vi "tvac_gui_v3.vi"() -> ()   [LabVIEW 2017]
uses:
  <vilib>/httpClient/ClientHandle.ctl
  msg7171_linux.llb/send single message.vi
  <vilib>/httpClient/POSTBuffer.vi
  <vilib>/httpClient/LabVIEWHTTPClient.lvlib
panel:
  in  "index (col)":i32
  in  "alarm":i32
  in  "NumberTCs":i32=10
  in  "Tab Control":enum32{"Page 1", "Page 2"}(tab)
  in  "Zone 1":T1 {"Ring" items=["Average", "Maximum", "Minimum", ""]}
  in  "Graphing Selection":u16(ring) items=["User Selection", "Graph All Thermocouples", "Clear Graph"]
  in  "Time Scale":u16(ring) items=["Minutes", "Hours", "Seconds"]
  out "Waveform Chart":waveform(dbl)[](graph)
  out "Thermocouples":T2(array[cluster])
  in  "exit":bool
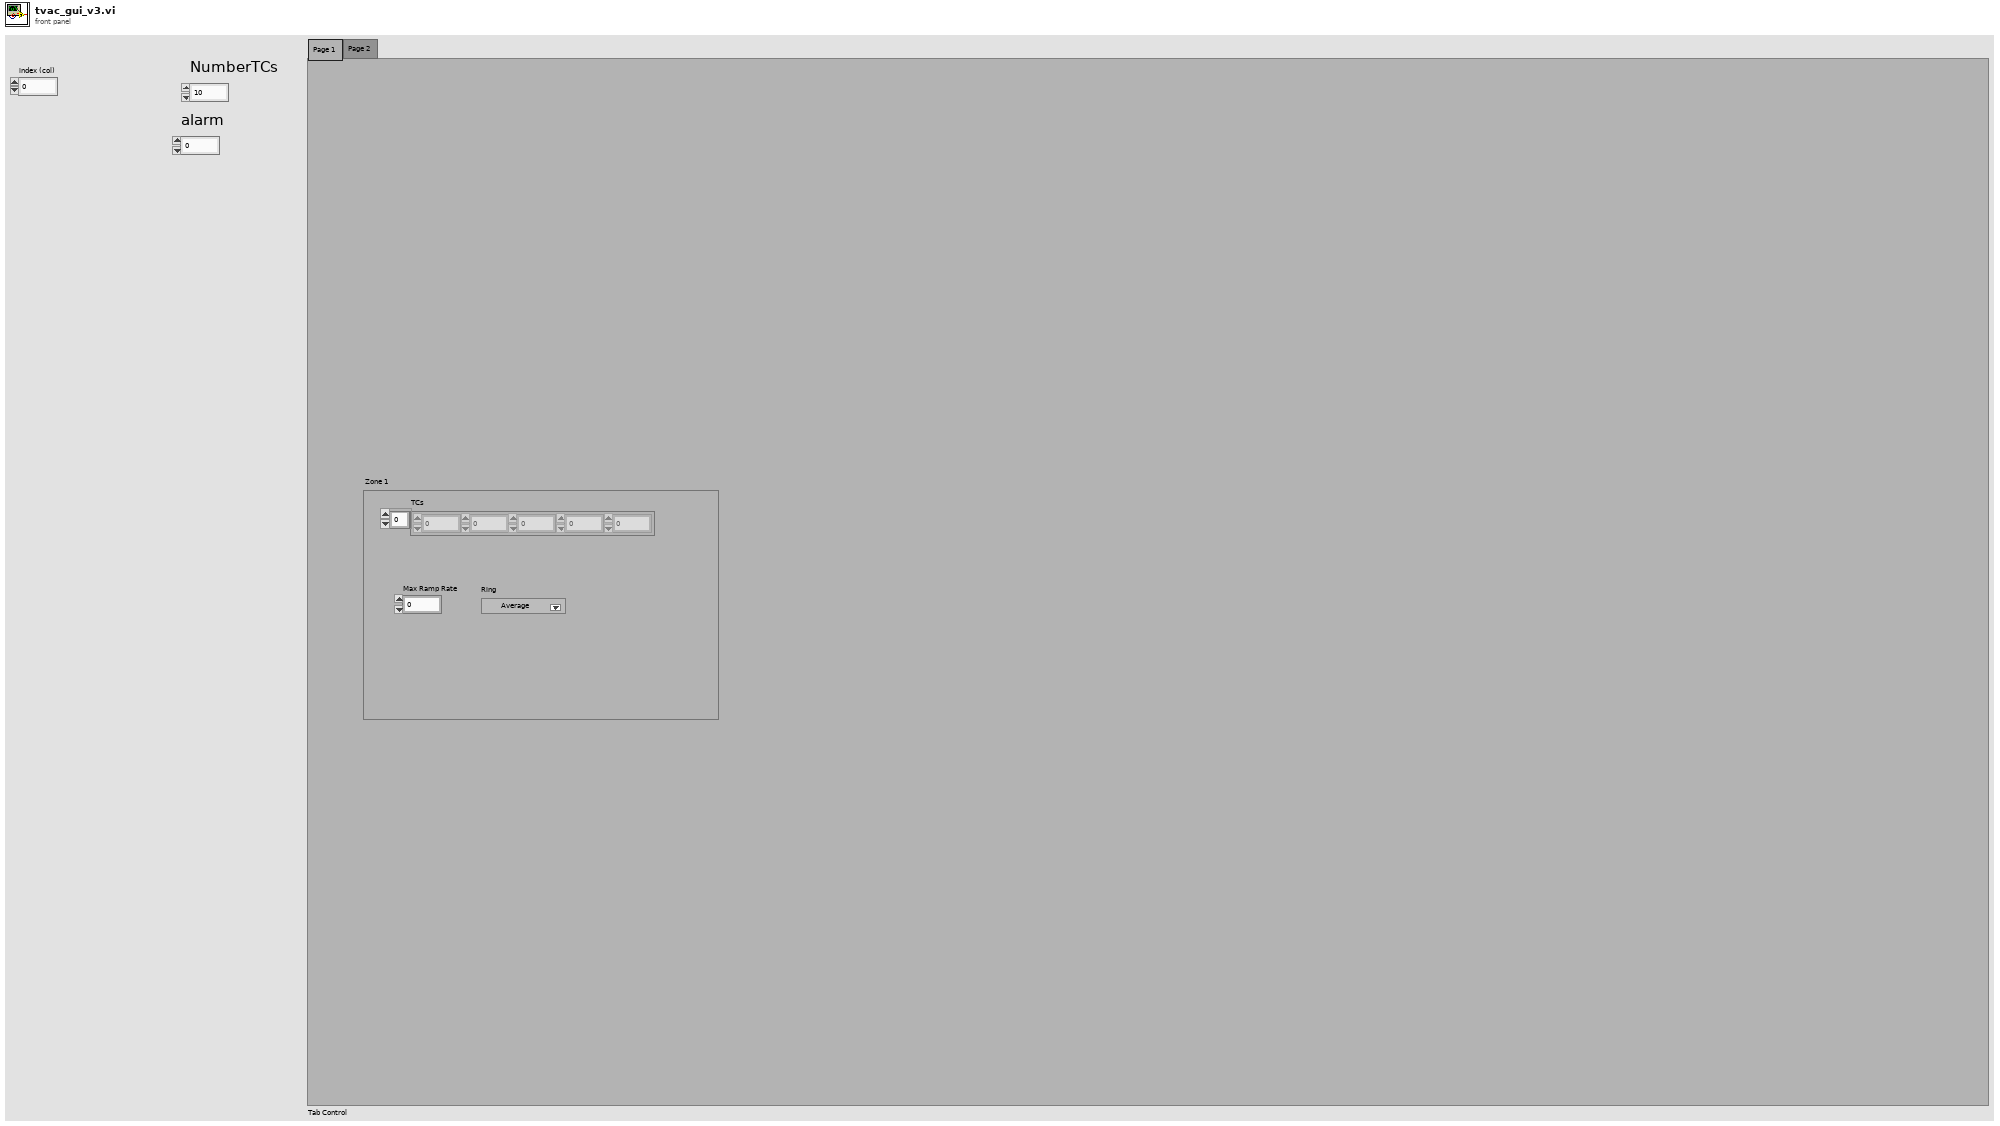
[diagram p1: front panel]
types:
  T1 = cluster{"Ring":u16, "Max Ramp Rate":dbl, "TCs":dbl[]}
  T2 = cluster{"TC Label":string, "Alarm Status":string, "Alarm Color":u32, "Temperature":string, "PlotColor":u32, "Graph On/Off":u32}[][]
  T3 = typedef "LabVIEWHTTPClient.lvlib/ClientHandle.ctl" = refnum<k1>
  T4 = cluster{"go":bool, "Http session":T3, "URL prefex":string}
  T5 = typedef "LVPoint32TypeDef.ctl" = cluster{"Horizontal":i32, "Vertical":i32}
  T6 = typedef "LVPositionTypeDef.ctl" = cluster{"Left":i32, "Top":i32}
  T7 = cluster{"TC Label":string, "Alarm Status":string, "Alarm Color":u32, "Temperature":string, "PlotColor":u32, "Graph On/Off":u32}
  T8 = typedef "LVRangeTypeDef.ctl" = cluster{"Minimum":dbl, "Maximum":dbl, "Increment":dbl, "Minor Increment":dbl, "Start":dbl}
  T9 = cluster{"time":string, "tcs":cluster{"thermocouple":i32, "time":i32, "temp":i32, "working":string, "alarm":i32}[]}
  T10 = cluster{"time":string, "tcs":cluster{"thermocouple":i32, "time":i32, "temp":i32, "working":i32, "alarm":i32}[]}
  T11 = cluster{"thermocouple":i32, "time":i32, "temp":i32, "working":i32, "alarm":i32}[]
  T12 = cluster{"thermocouple":i32, "time":i32, "temp":i32, "working":i32, "alarm":i32}
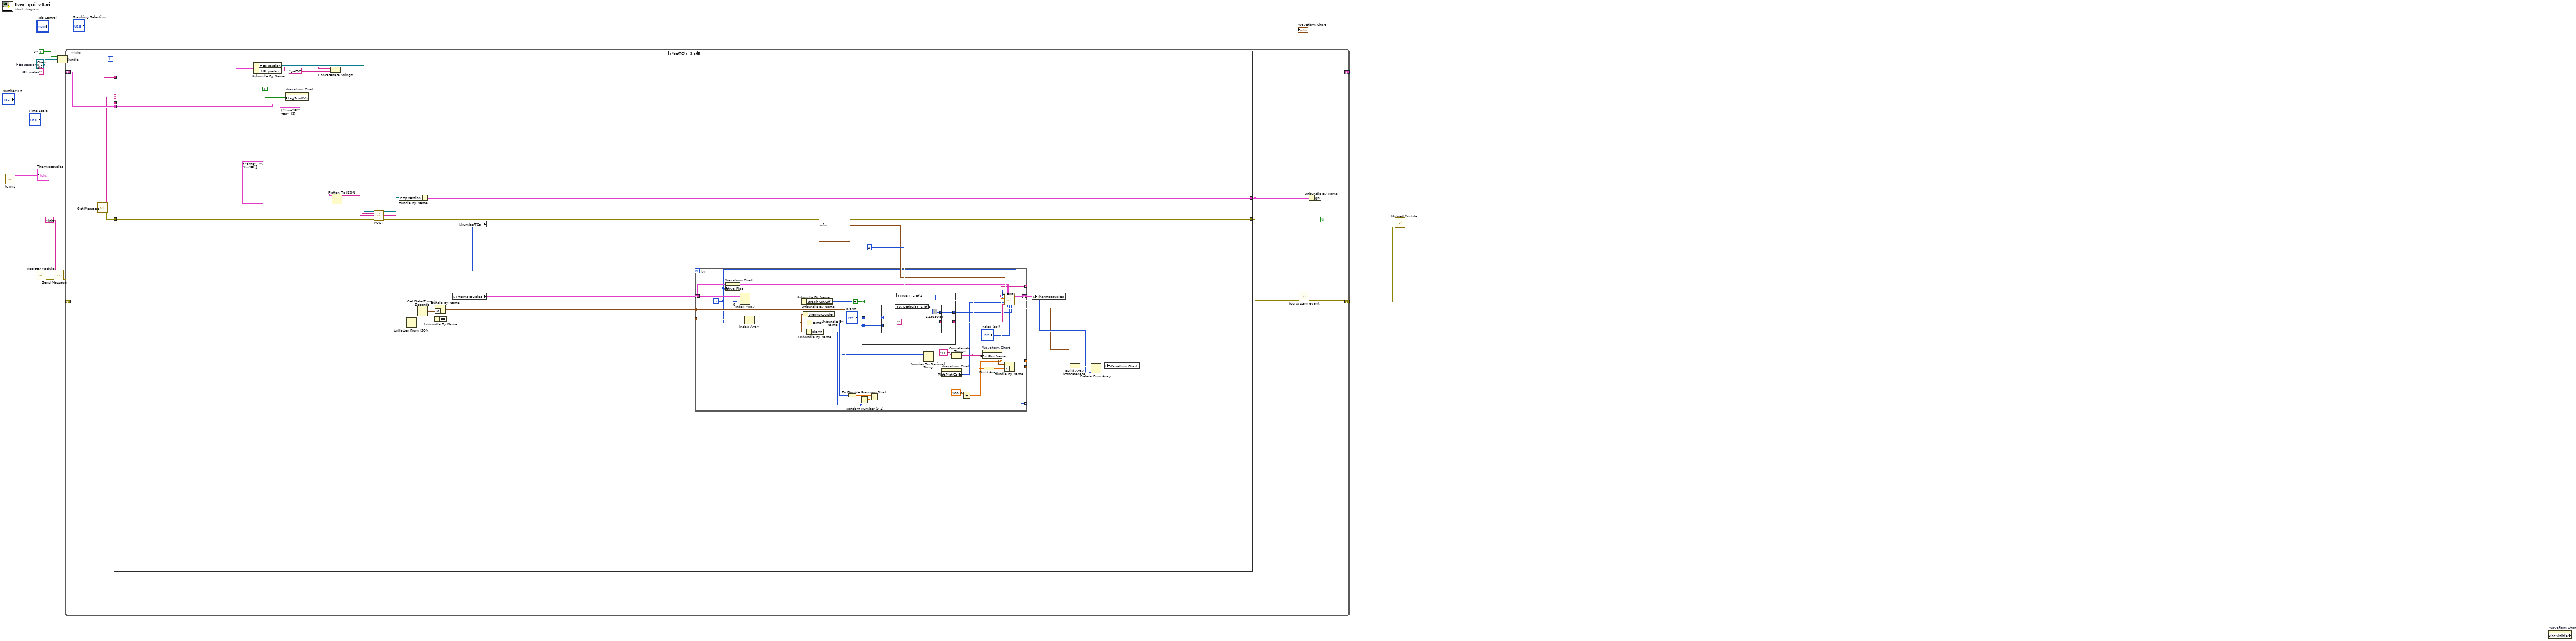
[diagram p0: block diagram]
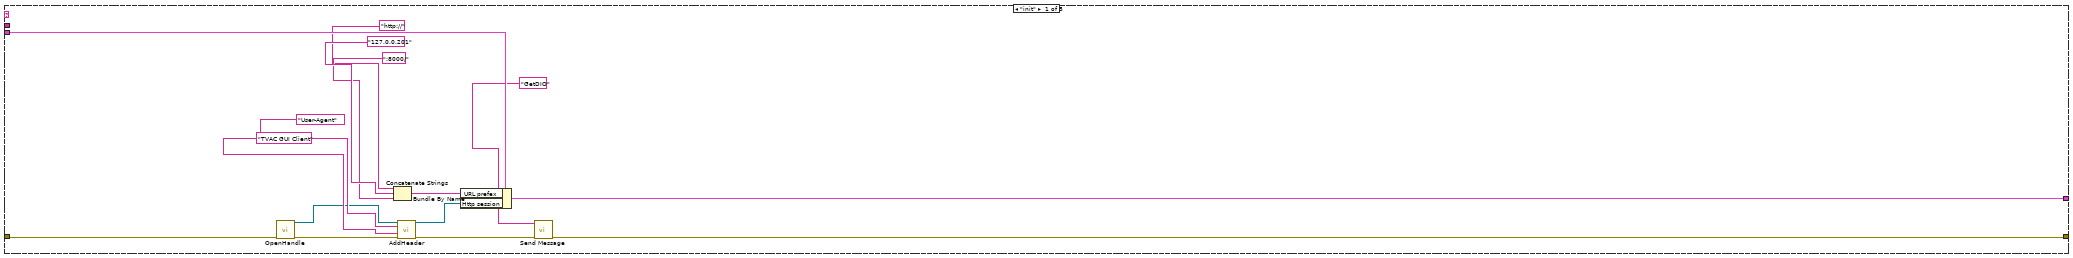
[diagram p2: hidden frame]
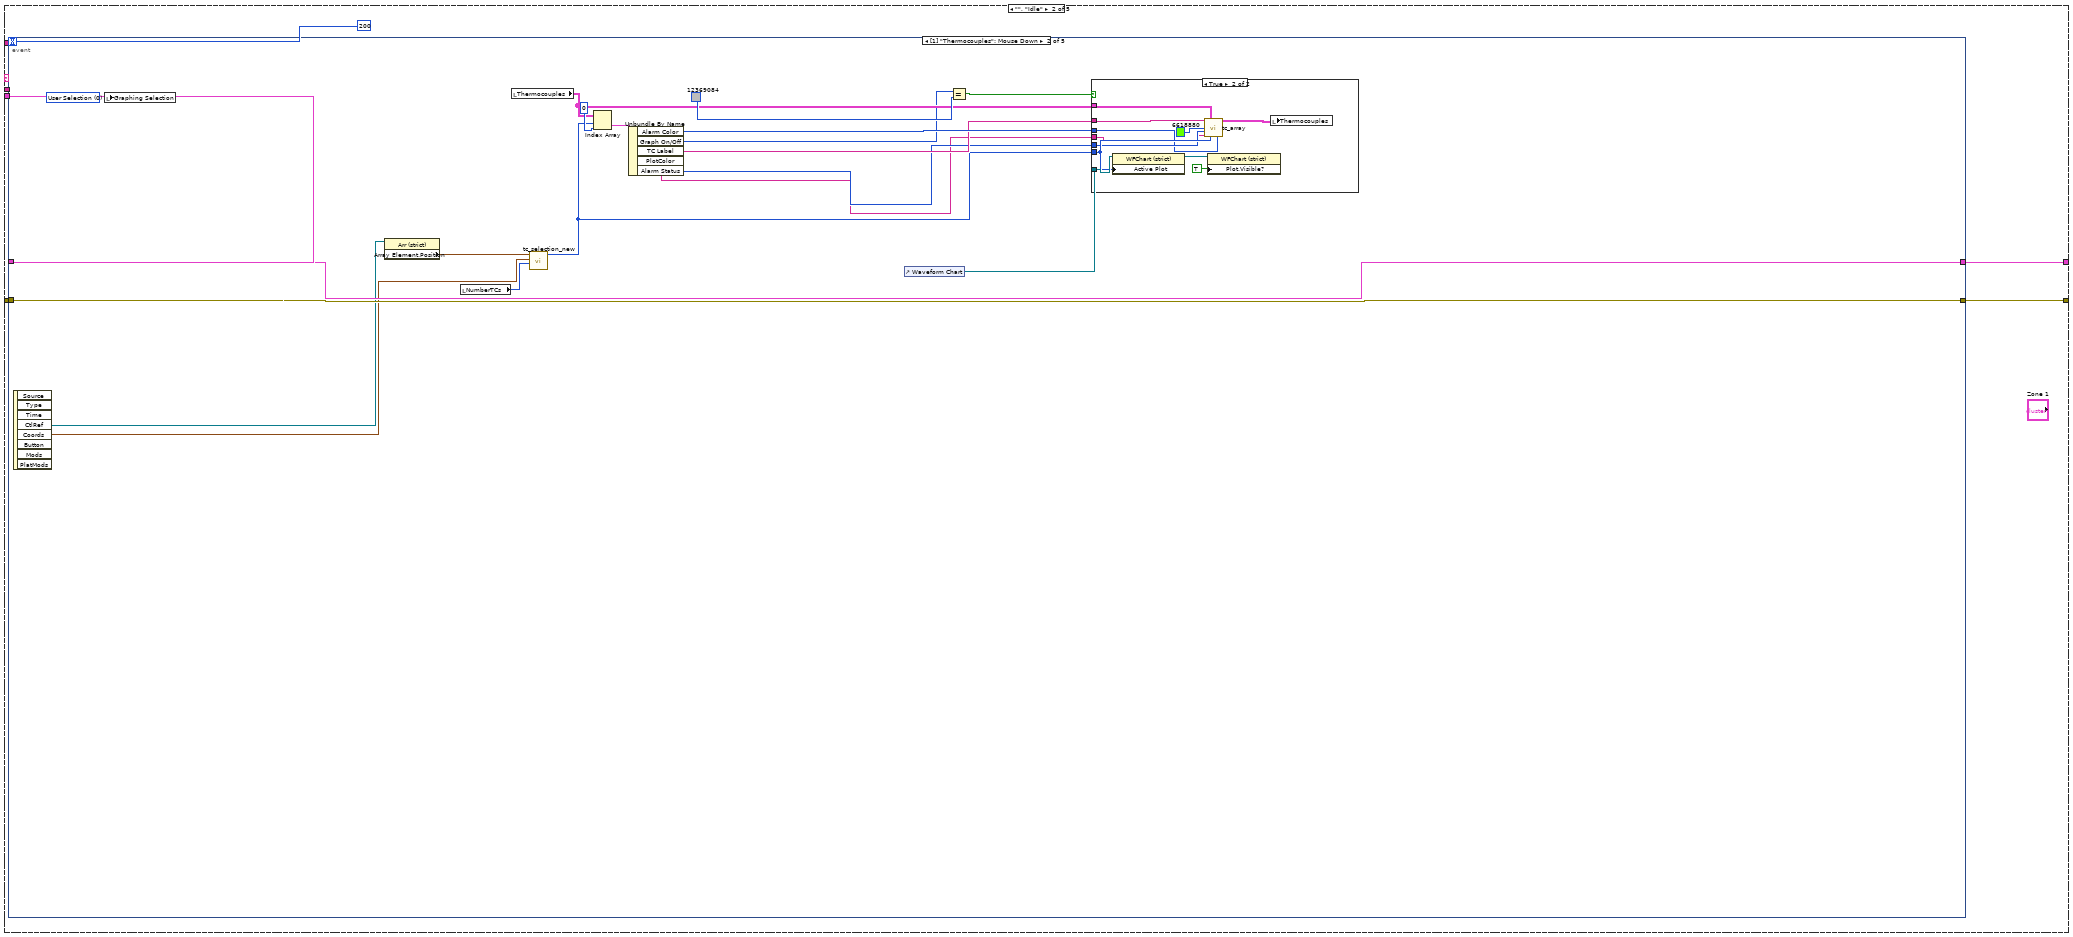
[diagram p3: hidden frame]
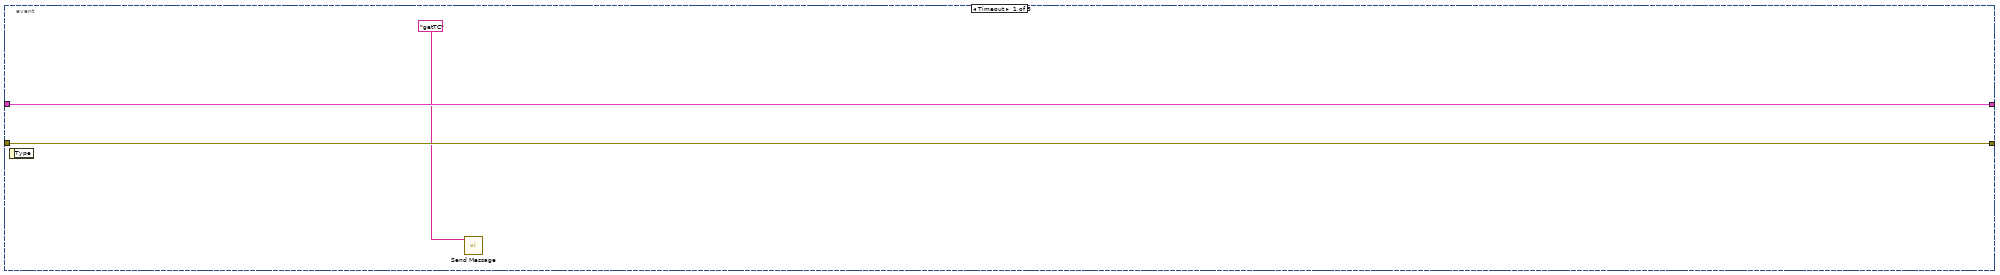
[diagram p4: hidden frame]
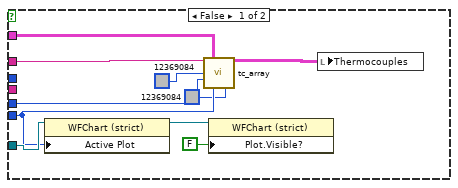
[diagram p5: hidden frame]
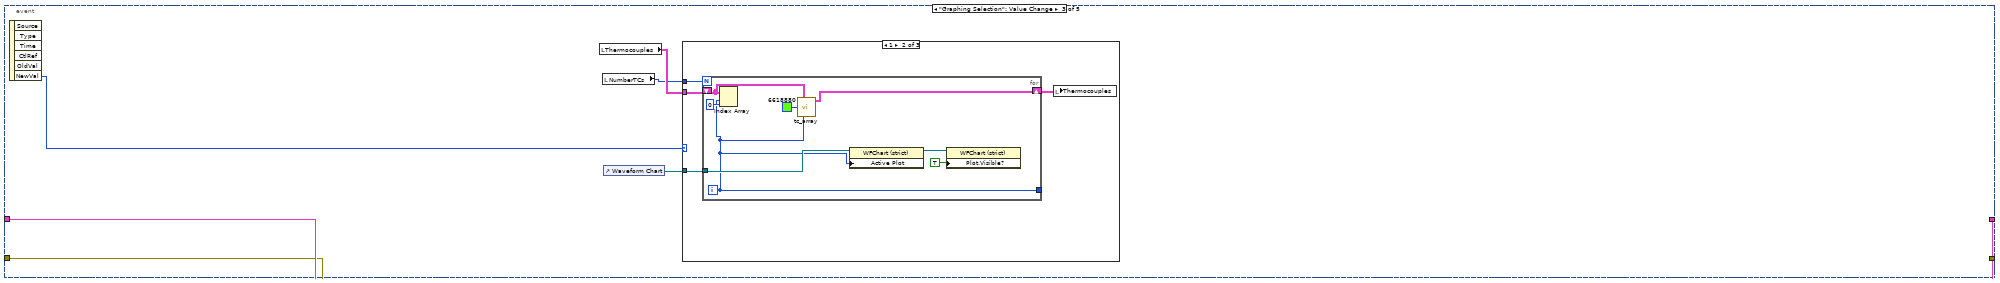
[diagram p6: hidden frame]
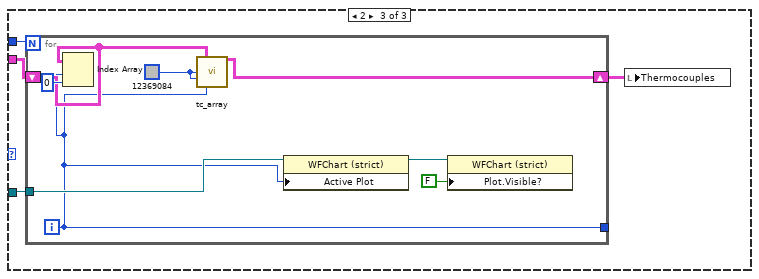
[diagram p8: hidden frame]
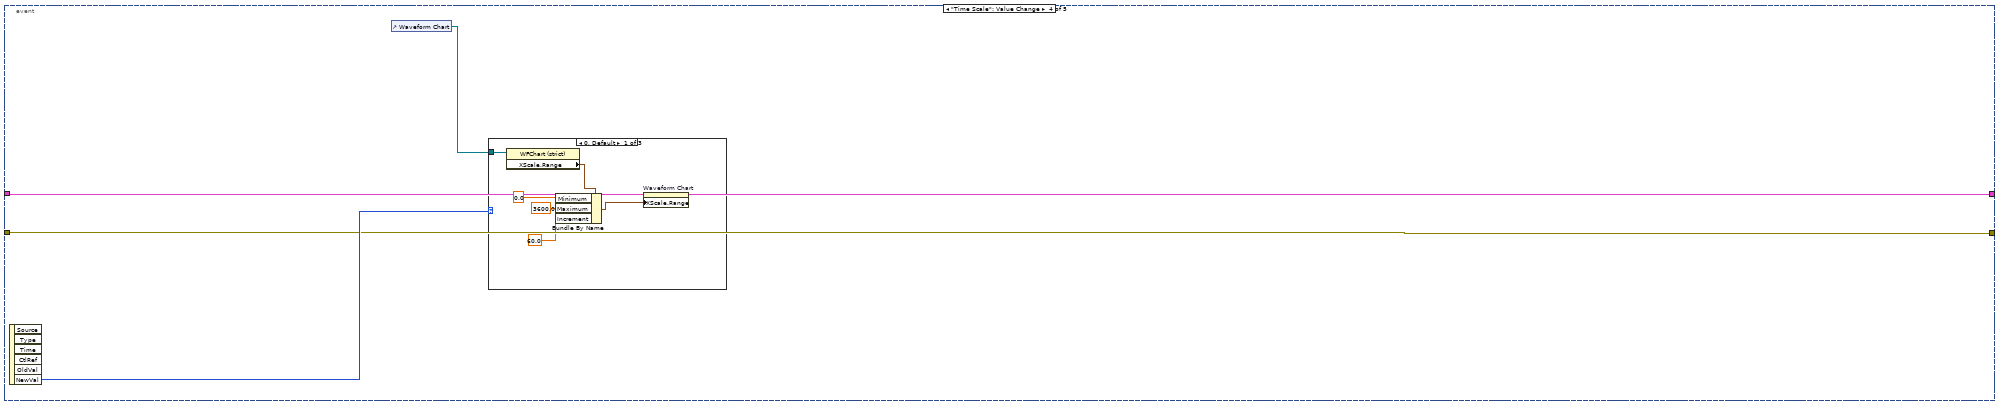
[diagram p9: hidden frame]
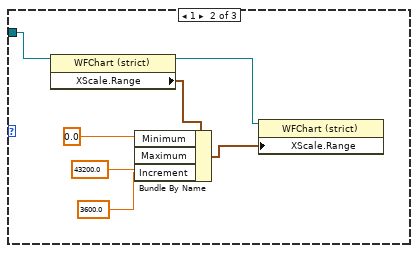
[diagram p10: hidden frame]
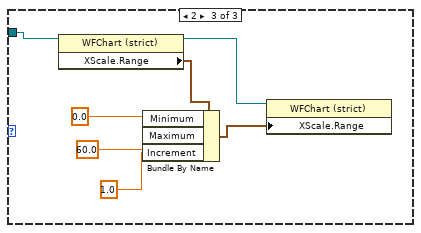
[diagram p11: hidden frame]
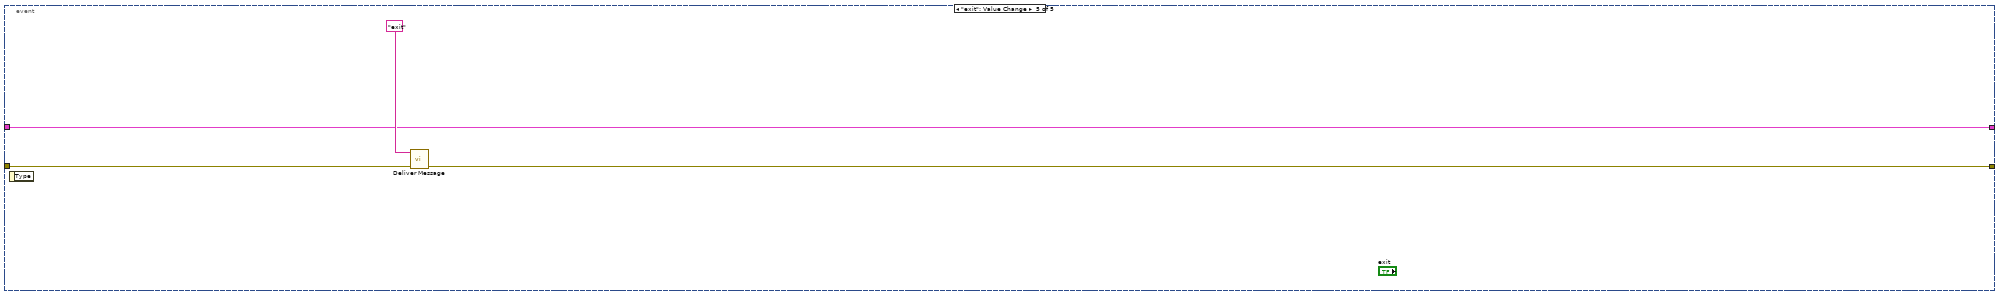
[diagram p12: hidden frame]
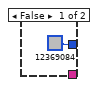
[diagram p13: hidden frame]
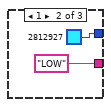
[diagram p14: hidden frame]
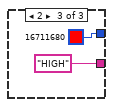
[diagram p15: hidden frame]
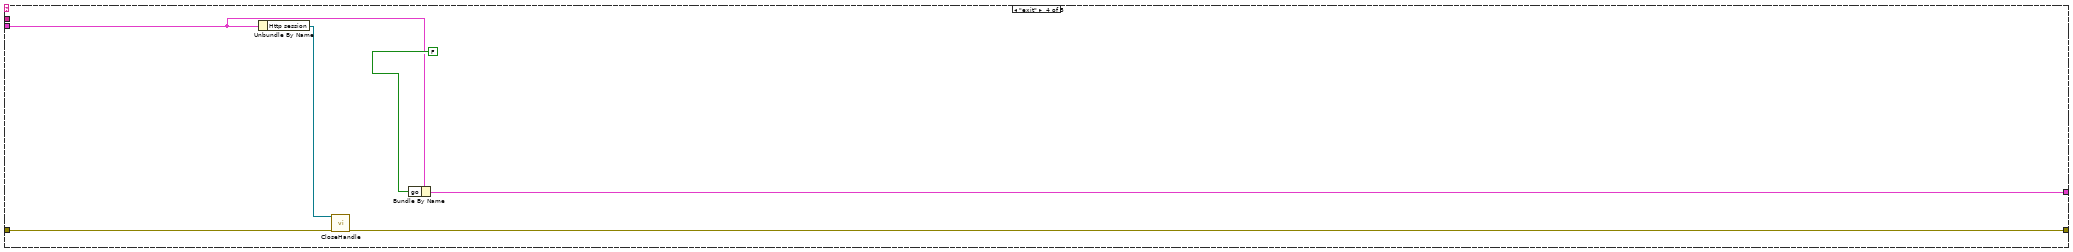
[diagram p16: hidden frame]
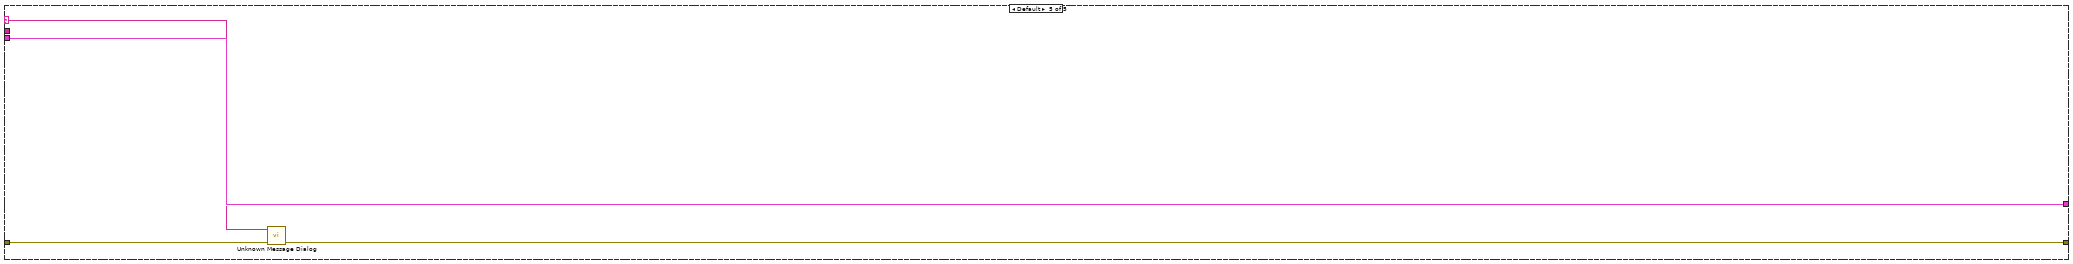
[diagram p17: hidden frame]
diagram:
  w5 = ""  # URL prefex
  w6 = T3 refnum  # Http session
  w7 = TRUE  # go
  n1 = call "tc_init.vi"() -> ("output array"=→"Thermocouples":T2)  [unwired: 15 in]
  n2 = call "Register Module.vi"() -> ("error out"=w3:errorcluster)  [unwired: 10 in, 1 out]
  n3 = call-poly "Send Message.vi"("error in (no error)"=w3, "event"="init") -> ("error out"=w2:errorcluster)  [unwired: 9 in]
  n4 = Bundle("go"=w7, "Http session"=w6, "URL prefex"=w5) -> (w9:T4)  [unwired: 1 in]
  n5 = while {
    shift-left: w9 -> [w16]
    shift-right: [w14] -> _
    shift-right: [w13] -> w8
    shift-left: w2 -> [w19]
    stop <- w10 continue-if-true
    n6 = call "Get Message.vi"("error in (no error)"=w19) -> ("error out"=w17:errorcluster, "event buffer"=w18:string, "event"=w15:string, "source"=w11:string)  [unwired: 7 in]
    n7 = case shown="\"getTC\"" w15 {
      selector: w15 -> [_ _ _ _ w212]
      tunnel: [w25 w36 w163 w210 w214] -> w14
      tunnel: w16 -> [w34 w35 w161 w205 w214]
      tunnel: w18 -> [_ _ _ _ _]
      tunnel: w17 -> [w29 w37 w165 w208 w213]
      tunnel: [w21 w39 w164 w207 w211] -> w12
      tunnel: w11 -> [_ _ _ _ _]
      frame "init" {
        n8 = call <vilib>:"OpenHandle.vi"("error in (no error)"=w29) -> ("client handle out"=w30:T3, "error out"=w33:errorcluster)  [unwired: 13 in]
        n9 = Concatenate Strings("http://" ("url"), "127.0.0.201" ("Address"), ":8000/" ("url")) -> (w24:string)
        n10 = call <vilib>:"AddHeader.vi"("client handle"=w30, "header"="User-Agent", "value"="TVAC GUI Client", "error in (no error)"=w33) -> ("client handle out"=w23:T3, "error out"=w22:errorcluster)  [unwired: 10 in]
        n11 = Bundle By Name(cluster=w34, "URL prefex"=w24, "Http session"=w23) -> (w25:T4)
        n12 = call-poly "Send Message.vi"("error in (no error)"=w22, "event"="GetDIO") -> ("error out"=w21:errorcluster)  [unwired: 9 in]
      }
      frame "", "Idle" {
        n13 = event shown="[1] \"Thermocouples\": Mouse Down" {
          selector: _ -> [_ _ _ _ _]
          dyn-events: _ -> [_ _ _ _ _]
          timeout: 200 ("milliseconds to wait") -> [_ _ _ _ _]
          tunnel: w37 -> [w41 w61 w87 w114 w140]
          tunnel: [w41 w61 w87 w114 w139] -> w39
          tunnel: [w42 w60 w88 w115 w137] -> w36
          tunnel: w35 -> [w42 w60 w88 w115 w137]
          event Timeout {
            n14 = event-data() -> ()  [unwired: 1 in, 1 out]
            n15 = call-poly "Send Message.vi"("event"="getTC") -> ()  [unwired: 10 in, 1 out]
          }
          event "Thermocouples": Mouse Down {
            w43 = u16 0 items=["User Selection", "Graph All Thermocouples", "Clear Graph"] ("Graphing Selection")
            n16 = event-data() -> ("CtlRef"=w57:refnum<vi>, "Coords"=w58:T5)  [unwired: 1 in, 6 out]
            n17 = local write "Graphing Selection"(w43) -> ()
            n18 = property class="Arr (strict)"(reference=w57) -> ("Array Element.Position"=w59:T6)  [unwired: 1 in, 2 out]
            n19 = local read "NumberTCs"() -> (w49:i32)
            n20 = local read "Thermocouples"() -> (w51:T2)
            n21 = call "tc_selection_new.vi"("Numeric 2"=w49, "Coords"=w58, "Position"=w59) -> ("Numeric"=w45:i32)  [unwired: 8 in]
            n22 = Index Array(array=w51, index (row)=w45, index (col)=0 ("disabled index (col)")) -> (element=w54:T7)
            n23 = Unbundle By Name(w54) -> ("Alarm Color"=w50:u32, "Graph On/Off"=w48:u32, "TC Label"=w47:string, "PlotColor"=w46:u32, "Alarm Status"=w44:string)
            n24 = control-ref of="Waveform Chart"() -> (w52:refnum<vi>)
            n25 = Equal?(x=w48, y=u32 12369084) -> (x = y?=w53:bool)
            n26 = case shown="True" w53 {
              tunnel: w45 -> [w63 w75]
              tunnel: w52 -> [w69 w80]
              tunnel: w51 -> [w65 w77]
              tunnel: w50 -> [_ w72]
              tunnel: w47 -> [w67 w79]
              tunnel: w46 -> [w64 w74]
              tunnel: w44 -> [_ w73]
              frame False {
                n27 = property on="Property Node" class="WFChart (strict)"(reference=w69, "Active Plot"=w63) -> (reference out=w70:refnum<vi>)  [unwired: 1 in, 1 out]
                n28 = call "tc_array.vi"("TC Label"=w67, "output array 2"=w65, "Graph ON/OFF"=u32 12369084, "Plot Color"=w64, "index (row)"=w63, "AlarmColor"=u32 12369084) -> ("output array"=w66:T2)  [unwired: 9 in]
                n29 = property class="WFChart (strict)"(reference=w70, "Plot.Visible?"=FALSE ("Plot.Visible")) -> ()  [unwired: 1 in, 2 out]
                n30 = local write "Thermocouples"(w66) -> ()
              }
              frame True {
                n31 = property class="WFChart (strict)"(reference=w80, "Active Plot"=w75) -> (reference out=w81:refnum<vi>)  [unwired: 1 in, 1 out]
                n32 = call "tc_array.vi"("TC Label"=w79, "output array 2"=w77, "Graph ON/OFF"=u32 6618880, "Plot Color"=w74, "Alarm String"=w73, "index (row)"=w75, "AlarmColor"=w72) -> ("output array"=w76:T2)  [unwired: 8 in]
                n33 = property class="WFChart (strict)"(reference=w81, "Plot.Visible?"=TRUE ("Plot.Visible")) -> ()  [unwired: 1 in, 2 out]
                n34 = local write "Thermocouples"(w76) -> ()
              }
            }
          }
          event "Graphing Selection": Value Change {
            n35 = event-data() -> ("NewVal"=w83:u16)  [unwired: 1 in, 5 out]
            n36 = local read "Thermocouples"() -> (w86:T2)
            n37 = local read "NumberTCs"() -> (w84:i32)
            n38 = control-ref of="Waveform Chart"() -> (w85:refnum<vi>)
            n39 = case shown="1" w83 {
              tunnel: w86 -> [_ w92 w103]
              tunnel: w85 -> [_ w91 w102]
              tunnel: w84 -> [_ w90 w104]
              frame 0, Default {
              }
              frame 1 {
                n40 = for {
                  N: w90 -> [_]
                  tunnel: w91 -> [w97]
                  tunnel: [w96] -> _
                  shift-right: [w94] -> w89
                  shift-left: w92 -> [w95]
                  i -> [w96]
                  n41 = Index Array(array=w95, index (row)=w96, index (col)=0 ("disabled index (col)")) -> ()  [unwired: 1 out]
                  n42 = call "tc_array.vi"("output array 2"=w95, "Graph ON/OFF"=u32 6618880, "index (row)"=w96) -> ("output array"=w94:T2)  [unwired: 12 in]
                  n43 = property class="WFChart (strict)"(reference=w97, "Active Plot"=w96) -> (reference out=w99:refnum<vi>)  [unwired: 1 in, 1 out]
                  n44 = property class="WFChart (strict)"(reference=w99, "Plot.Visible?"=TRUE ("Plot.Visible")) -> ()  [unwired: 1 in, 2 out]
                }
                n45 = local write "Thermocouples"(w89) -> ()
              }
              frame 2 {
                n46 = for {
                  N: w104 -> [_]
                  tunnel: w102 -> [w109]
                  tunnel: [w107] -> _
                  shift-right: [w105] -> w101
                  shift-left: w103 -> [w108]
                  i -> [w107]
                  w106 = u32 12369084
                  n47 = Index Array(array=w108, index (row)=w107, index (col)=0 ("disabled index (col)")) -> ()  [unwired: 1 out]
                  n48 = call "tc_array.vi"("output array 2"=w108, "Graph ON/OFF"=w106, "Plot Color"=w106, "index (row)"=w107) -> ("output array"=w105:T2)  [unwired: 11 in]
                  n49 = property class="WFChart (strict)"(reference=w109, "Active Plot"=w107) -> (reference out=w111:refnum<vi>)  [unwired: 1 in, 1 out]
                  n50 = property class="WFChart (strict)"(reference=w111, "Plot.Visible?"=FALSE ("Plot.Visible")) -> ()  [unwired: 1 in, 2 out]
                }
                n51 = local write "Thermocouples"(w101) -> ()
              }
            }
          }
          event "Time Scale": Value Change {
            n52 = event-data() -> ("NewVal"=w116:u16)  [unwired: 1 in, 5 out]
            n53 = control-ref of="Waveform Chart"() -> (w113:refnum<vi>)
            n54 = case shown="0, Default" w116 {
              tunnel: w113 -> [w120 w124 w131]
              frame 0, Default {
                n55 = property on="Property Node" class="WFChart (strict)"(reference=w120) -> ("XScale.Range"=w122:T8)  [unwired: 1 in, 2 out]
                n56 = Bundle By Name(cluster=w122, "Minimum"=0.0, "Maximum"=3600.0, "Increment"=60.0) -> (w121:T8)
                n57 = property on="Waveform Chart" class="WFChart (strict)"("XScale.Range"=w121) -> ()  [unwired: 2 in, 2 out]
              }
              frame 1 {
                n58 = property on="Property Node" class="WFChart (strict)"(reference=w124) -> (reference out=w123:refnum<vi>, "XScale.Range"=w129:T8)  [unwired: 1 in, 1 out]
                n59 = Bundle By Name(cluster=w129, "Minimum"=0.0, "Maximum"=43200.0, "Increment"=3600.0) -> (w125:T8)
                n60 = property on="Property Node" class="WFChart (strict)"(reference=w123, "XScale.Range"=w125) -> ()  [unwired: 1 in, 2 out]
              }
              frame 2 {
                n61 = property on="Property Node" class="WFChart (strict)"(reference=w131) -> (reference out=w130:refnum<vi>, "XScale.Range"=w136:T8)  [unwired: 1 in, 1 out]
                n62 = Bundle By Name(cluster=w136, "Minimum"=0.0, "Maximum"=60.0, "Increment"=1.0) -> (w132:T8)
                n63 = property on="Property Node" class="WFChart (strict)"(reference=w130, "XScale.Range"=w132) -> ()  [unwired: 1 in, 2 out]
              }
            }
          }
          event "exit": Value Change {
            n64 = event-data() -> ()  [unwired: 1 in, 1 out]
            n65 = call "Deliver Message.vi"("error in (no error)"=w140, "event"="exit") -> ("error out"=w139:errorcluster)  [unwired: 9 in]
          }
        }
      }
      frame "getTC" {
        (unwired) T9 {"time"="", "tcs"=[]}
        w141 = T10 {"time"="", "tcs"=[]} ("Cluster")
        n66 = Unbundle By Name(w161) -> ("Http session"=w160:T3, "URL prefex"=w158:string)
        n67 = property on="Waveform Chart" class="WFChart (strict)"("LegScrollVis"=TRUE ("Legend:Scrollbar Visible")) -> ()  [unwired: 2 in, 2 out]
        n68 = Concatenate Strings(w158, "getTC" ("url")) -> (w159:string)
        n69 = Flatten To JSON(anything=w141) -> (JSON string=w156:string)  [unwired: 2 in, 1 out]
        n70 = call-poly <vilib>:"POST.vi"("client handle"=w160, "url"=w159, "buffer"=w156, "error in (no error)"=w165) -> ("client handle out"=w162:T3, "body"=w155:string, "error out"=w164:errorcluster)  [unwired: 8 in, 1 out]
        n71 = Bundle By Name(cluster=w161, "Http session"=w162) -> (w163:T4)
        n72 = Unflatten From JSON(JSON string=w155, type and defaults=w141) -> (value=w154:T10)  [unwired: 5 in, 1 out]
        n73 = Get Date/Time In Seconds() -> (seconds since 1Jan1904=w150:timestamp)
        n74 = Unbundle By Name(w154) -> ("tcs"=w153:T11)
        n75 = Bundle By Name("t0"=w150) -> (w149:waveform(dbl))  [unwired: 1 in]
        n76 = local read "Thermocouples"() -> (w145:T2)
        n77 = local read "NumberTCs"() -> (w142:i32)
        n78 = for {
          N: w142 -> [_]
          tunnel: w153 -> [w193]
          tunnel: w149 -> [w191]
          tunnel: [w192] -> w148 mode=indexing
          tunnel: [w174] -> _ mode=indexing
          tunnel: [w173] -> _ mode=indexing
          tunnel: [w176] -> _ mode=indexing
          shift-right: [w175] -> w146
          shift-left: w145 -> [w172]
          i -> [w166]
          n79 = property on="Waveform Chart" class="WFChart (strict)"("Active Plot"=w166) -> ()  [unwired: 2 in, 2 out]
          n80 = Index Array(array=w172, index (row)=w166, index (col)=0 ("disabled index (col)")) -> (element=w179:T7)
          n81 = Index Array(array=w193, index=w166) -> (element=w183:T12)
          n82 = Unbundle By Name(w179) -> ("Graph On/Off"=w169:u32)
          n83 = Unbundle By Name(w183) -> ("thermocouple"=w189:i32)
          n84 = Unbundle By Name(w183) -> ("alarm"=w176:i32)
          n85 = Unbundle By Name(w183) -> ("temp"=w187:i32)
          n86 = To Double Precision Float(number=w187) -> (double precision float=w184:dbl)
          n87 = Random Number (0-1)() -> (number: 0 to 1=w185:dbl)
          n88 = case shown="True" TRUE {
            tunnel: [_ w198] -> w171
            tunnel: "alarm" -> [_ w197]
            tunnel: w176 -> [_ w196]
            tunnel: [u32 12369084 w195] -> w168
            frame False {
            }
            frame True {
              n89 = case shown="0, Default" w197 {
                tunnel: ["" "LOW" "HIGH"] -> w198
                tunnel: w196 -> [_ _ _]
                tunnel: [u32 12369084 u32 2812927 u32 16711680] -> w195
                frame 0, Default {
                }
                frame 1 {
                }
                frame 2 {
                }
              }
            }
          }
          n90 = Add(x=w184, y=w185) -> (x+y=w181:dbl)
          n91 = Number To Decimal String(number=w189) -> (decimal integer string=w190:string)  [unwired: 1 in]
          n92 = property on="Waveform Chart" class="WFChart (strict)"() -> ("Plot.Plot Color"=w170:u32)  [unwired: 2 in, 2 out]
          n93 = Concatenate Strings("TC " ("string"), w190) -> (w173:string)
          n94 = Add(x=100.0, y=w181) -> (x+y=w174:dbl)
          n95 = property on="Waveform Chart" class="WFChart (strict)"("Plot.Plot Name"=w173) -> ()  [unwired: 2 in, 2 out]
          n96 = Build Array(w174) -> (w186:dbl[])
          n97 = call "tc_array.vi"("TC Label"=w173, "output array 2"=w172, "Temperature"=w174, "Graph ON/OFF"=w169, "Plot Color"=w170, "Alarm String"=w171, "index (row)"=w166, "index (col)"="index (col)", "AlarmColor"=w168) -> ("output array"=w175:T2)  [unwired: 6 in]
          n98 = Bundle By Name(cluster=w191, "Y"=w186) -> (w192:waveform(dbl))
        }
        n99 = local write "Thermocouples"(w146) -> ()
        n100 = Build Array (concatenate)(waveform(dbl) {"t0"=timestamp(0 s since 1904-01-01), "dt"=1.0, "Y"=[]} ("element"), w148) -> (w152:waveform(dbl)[])
        n101 = Delete From Array(array=w152, index=0) -> (array with subset deleted=w143:waveform(dbl)[])  [unwired: 1 in, 1 out]
        n102 = local write "Waveform Chart"(w143) -> ()
      }
      frame "exit" {
        n103 = Unbundle By Name(w205) -> ("Http session"=w206:T3)
        n104 = call <vilib>:"CloseHandle.vi"("client handle"=w206, "error in (no error)"=w208) -> ("error out"=w207:errorcluster)  [unwired: 13 in]
        n105 = Bundle By Name(cluster=w205, "go"=FALSE ("Bundle Element")) -> (w210:T4)
      }
      frame Default {
        n106 = call "Unknown Message Dialog.vi"("error in (no error)"=w213, "event name"=w212) -> ("error out"=w211:errorcluster)  [unwired: 9 in]
      }
    }
    n107 = call "log system event.vi"("error in (no error)"=w12) -> ("error out"=w13:errorcluster)  [unwired: 9 in, 1 out]
    n108 = Unbundle By Name(w14) -> ("go"=w10:bool)
  }
  n109 = call "Unload Module.vi"("error in (no error)"=w8) -> ()  [unwired: 10 in, 1 out]
  n110 = property on="Waveform Chart" class="WFChart (strict)" props=["Plot", "Visible?"]() -> ()  [unwired: 2 in, 3 out]
